vi "写入控制命令.vi"(8 "error in (no error)":errorcluster, 11 "命令":T1(ring)) -> (0 "error out":errorcluster)   [LabVIEW 2016, in "一代CodMn.lvlib"]
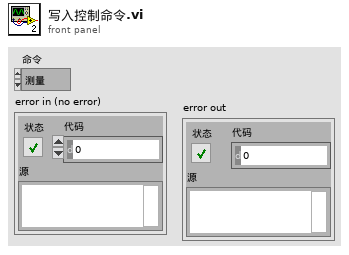
[diagram p1: front panel]
types:
  T1 = enum16{"测量", "校零", "校标", "填充管路", "外部停止", "连续测量", "空白测量", "标样测量", "故障状态清除"}
  T2 = enum16{"open", "close", "readHR", "writeHR", "readCoil", "writeCoil"}
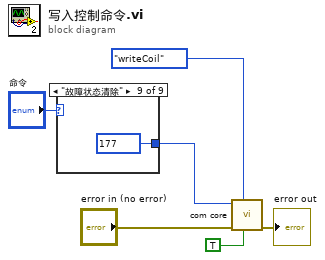
[diagram p0: block diagram]
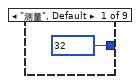
[diagram p2: hidden frame]
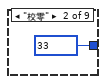
[diagram p3: hidden frame]
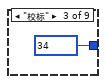
[diagram p4: hidden frame]
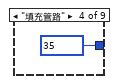
[diagram p5: hidden frame]
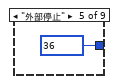
[diagram p6: hidden frame]
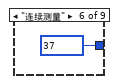
[diagram p7: hidden frame]
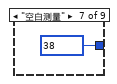
[diagram p8: hidden frame]
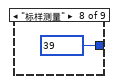
[diagram p9: hidden frame]
diagram:
  n1 = case shown="\"故障状态清除\"" "命令" {
    tunnel: [u16 32 ("starting address") u16 33 ("starting address") u16 34 ("starting address") u16 35 ("starting address") u16 36 ("starting address") u16 37 ("starting address") u16 38 ("starting address") u16 39 ("starting address") u16 177 ("starting address")] -> w4
    frame "测量", Default {
    }
    frame "校零" {
    }
    frame "校标" {
    }
    frame "填充管路" {
    }
    frame "外部停止" {
    }
    frame "连续测量" {
    }
    frame "空白测量" {
    }
    frame "标样测量" {
    }
    frame "故障状态清除" {
    }
  }
  n2 = call "com core.vi"("Coil value"=TRUE, "功能"=T2."writeCoil", "error in (no error)"="error in (no error)", "starting address"=w4) -> ("error out"=→"error out":errorcluster)  [unwired: 5 in, 2 out]
